vi "Test XML Schema.vi"() -> ()   [LabVIEW 2014]
uses:
  <vilib>/xml/Close Reference(Node).vi
  <vilib>/xml/NI_XML.lvlib
  <resource>/objmgr/DOMUserDefRef.rc
panel:
  out "error out":errorcluster
  out "XML":string
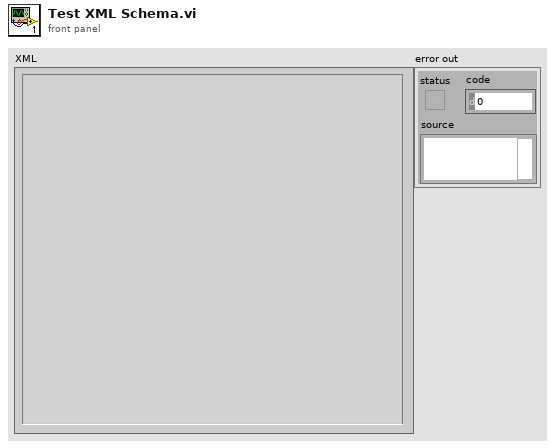
[diagram p1: front panel]
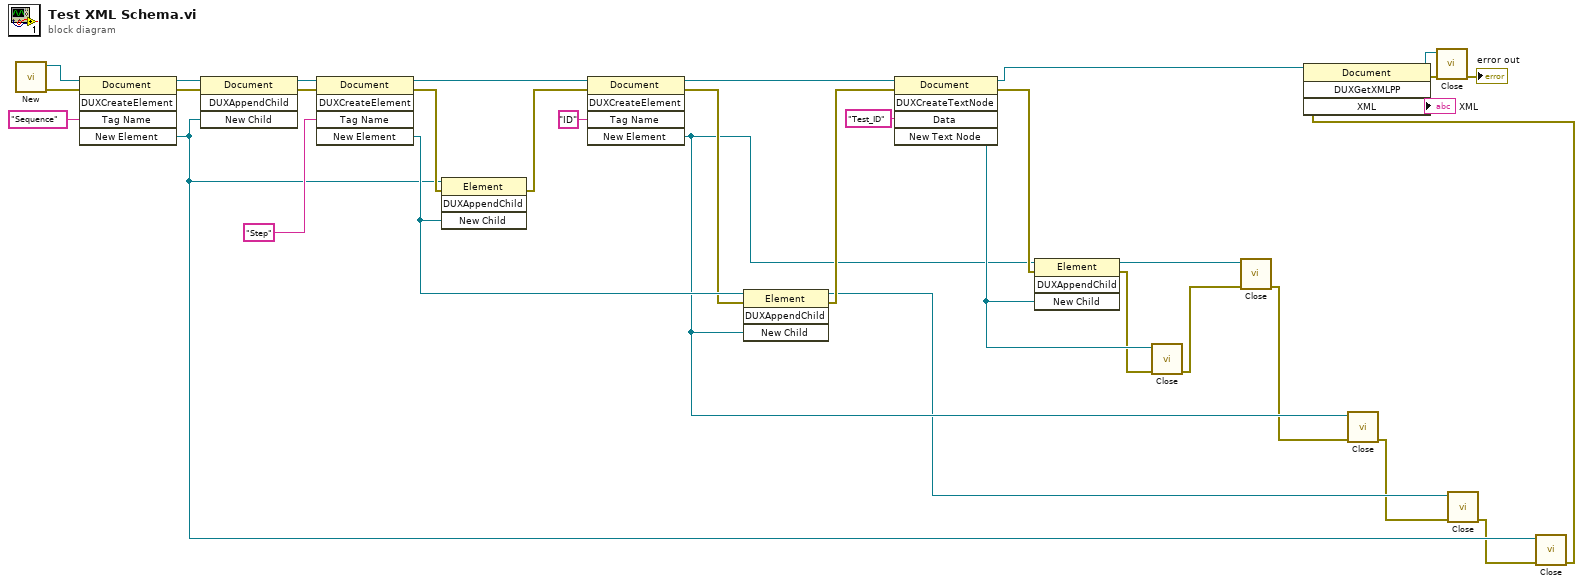
[diagram p0: block diagram]
diagram:
  n1 = call <vilib>:"New.vi"() -> ("error out"=w32:errorcluster, "DOM document out"=w30:refnum<k20>)  [unwired: 1 in, 7 out]
  n2 = invoke class="Document" method="DUXCreateElement"(reference=w30, error in=w32, "Tag Name"="Sequence" ("Qualified Name")) -> (reference out=w33:refnum<k20>, error out=w31:errorcluster, "New Element"=w5:refnum<k20>)  [unwired: 2 in, 2 out]
  n3 = invoke class="Document" method="DUXAppendChild"(reference=w33, error in=w31, "New Child"=w5) -> (reference out=w29:refnum<k20>, error out=w27:errorcluster)  [unwired: 1 in, 2 out]
  n4 = invoke class="Document" method="DUXCreateElement"(reference=w29, error in=w27, "Tag Name"="Step") -> (reference out=w26:refnum<k20>, error out=w18:errorcluster, "New Element"=w16:refnum<k20>)  [unwired: 2 in, 2 out]
  n5 = invoke class="Element" method="DUXAppendChild"(reference=w5, error in=w18, "New Child"=w16) -> (error out=w17:errorcluster)  [unwired: 1 in, 3 out]
  n6 = invoke class="Document" method="DUXCreateElement"(reference=w26, error in=w17, "Tag Name"="ID") -> (reference out=w24:refnum<k20>, error out=w15:errorcluster, "New Element"=w9:refnum<k20>)  [unwired: 2 in, 2 out]
  n7 = invoke class="Element" method="DUXAppendChild"(reference=w16, error in=w15, "New Child"=w9) -> (reference out=w7:refnum<k20>, error out=w14:errorcluster)  [unwired: 1 in, 2 out]
  n8 = invoke class="Document" method="DUXCreateTextNode"(reference=w24, error in=w14, "Data"="Test_ID") -> (reference out=w2:refnum<k20>, error out=w13:errorcluster, "New Text Node"=w12:refnum<k20>)  [unwired: 2 in, 2 out]
  n9 = invoke class="Element" method="DUXAppendChild"(reference=w9, error in=w13, "New Child"=w12) -> (reference out=w22:refnum<k20>, error out=w11:errorcluster)  [unwired: 1 in, 2 out]
  n10 = call-poly <vilib>:"Close.vi"("error in (no error)"=w11, "node"=w12) -> ("error out"=w10:errorcluster)  [unwired: 7 out]
  n11 = call-poly <vilib>:"Close.vi"("error in (no error)"=w10, "node"=w22) -> ("error out"=w8:errorcluster)  [unwired: 7 out]
  n12 = call-poly <vilib>:"Close.vi"("error in (no error)"=w8, "node"=w9) -> ("error out"=w6:errorcluster)  [unwired: 7 out]
  n13 = call-poly <vilib>:"Close.vi"("error in (no error)"=w6, "node"=w7) -> ("error out"=w4:errorcluster)  [unwired: 7 out]
  n14 = call-poly <vilib>:"Close.vi"("error in (no error)"=w4, "node"=w5) -> ("error out"=w3:errorcluster)  [unwired: 7 out]
  n15 = invoke class="Document" method="DUXGetXMLPP"(reference=w2, error in=w3) -> (reference out=w21:refnum<k20>, error out=w20:errorcluster, "XML"=→"XML":string)  [unwired: 2 in, 1 out]
  n16 = call-poly <vilib>:"Close.vi"("error in (no error)"=w20, "node"=w21) -> ("error out"=→"error out":errorcluster)  [unwired: 7 out]
